vi "RPT Comaristion.vi"(10 "True":bool) -> (1 "Fail":bool)   [LabVIEW 2020]
uses:
  Galobal variable_TI.vi
  Project Setup/Globle Variable/GR_Servo.vi
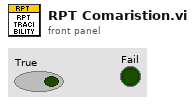
[diagram p1: front panel]
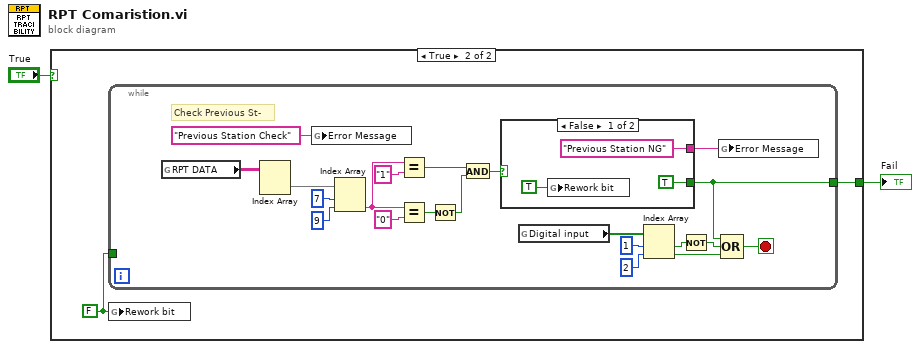
[diagram p0: block diagram]
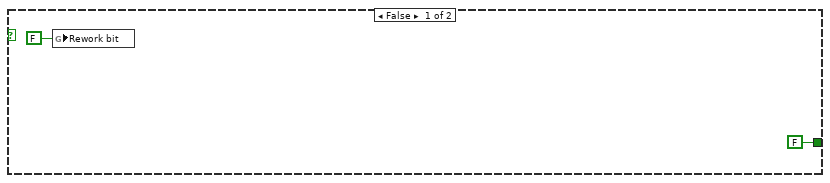
[diagram p2: hidden frame]
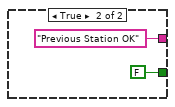
[diagram p3: hidden frame]
diagram:
  n1 = case shown="True" "True" {
    tunnel: [FALSE w6] -> w1
    frame False {
      n2 = global write "Galobal variable_TI.vi" "Rework bit"(FALSE ("Rework bit")) -> ()
    }
    frame True {
      w5 = FALSE ("Rework bit")
      n3 = while {
        tunnel: [w7] -> w6
        tunnel: w5 -> [_]
        stop <- w8 stop-if-true
        # "Check Previous St-"
        n4 = global read "GR_Servo.vi" "RPT DATA"() -> (w14:string[][])
        n5 = Index Array(array=w14) -> (element=w17:string[])  [unwired: 2 in]
        n6 = global write "GR_Servo.vi" "Error Message"("Previous Station Check") -> ()
        n7 = Index Array(array=w17, index #1=7 ("index"), index #2=9 ("index")) -> (element #2=w21:string)  [unwired: 1 out]
        n8 = Equal?(x=w21, y="1") -> (x = y?=w12:bool)
        n9 = Equal?(x=w21, y="0") -> (x = y?=w11:bool)
        n10 = Not(x=w11) -> (.not. x?=w10:bool)
        n11 = And(x=w12, y=w10) -> (x .and. y?=w9:bool)
        n12 = case shown="False" w9 {
          tunnel: ["Previous Station NG" "Previous Station OK"] -> w13
          tunnel: [TRUE FALSE] -> w7
          frame False {
            n13 = global write "Galobal variable_TI.vi" "Rework bit"(TRUE ("Rework bit")) -> ()
          }
          frame True {
          }
        }
        n14 = global read "Galobal variable_TI.vi" "Digital input"() -> (w27:bool[])
        n15 = Index Array(array=w27, index #1=1 ("index"), index #2=2 ("index")) -> (element #1=w24:bool, element #2=w22:bool)
        n16 = Not(x=w24) -> (.not. x?=w23:bool)
        n17 = global write "GR_Servo.vi" "Error Message"(w13) -> ()
        n18 = Compound Arithmetic op=OR(w7, w23, w22) -> (w8:bool)
      }
      n19 = global write "Galobal variable_TI.vi" "Rework bit"(w5) -> ()
    }
  }
  "Fail" <- w1
